vi "Save.vi"(0 "Digital in":refnum<vi>, 1 "new file path (Not A Path if cancelled) in":path, 2 "refnum in":refnum<file>, 5 "byte order (0:big-endian, network order)":T1(ring), 7 "Array":dbl[][](array[numeric]), 9 "Cluster":T2, 12 "Recording":bool, 13 "data":dbl[][](array[numeric]), 14 "Array 2":dbl[](array[numeric])) -> (4 "Byte Stream File out":refnum<file>, 6 "Save Path":path, 15 "new file path (Not A Path if cancelled)":path)   [LabVIEW 2018]
uses:
  <vilib>/Utility/file.llb/Write Delimited Spreadsheet (DBL).vi
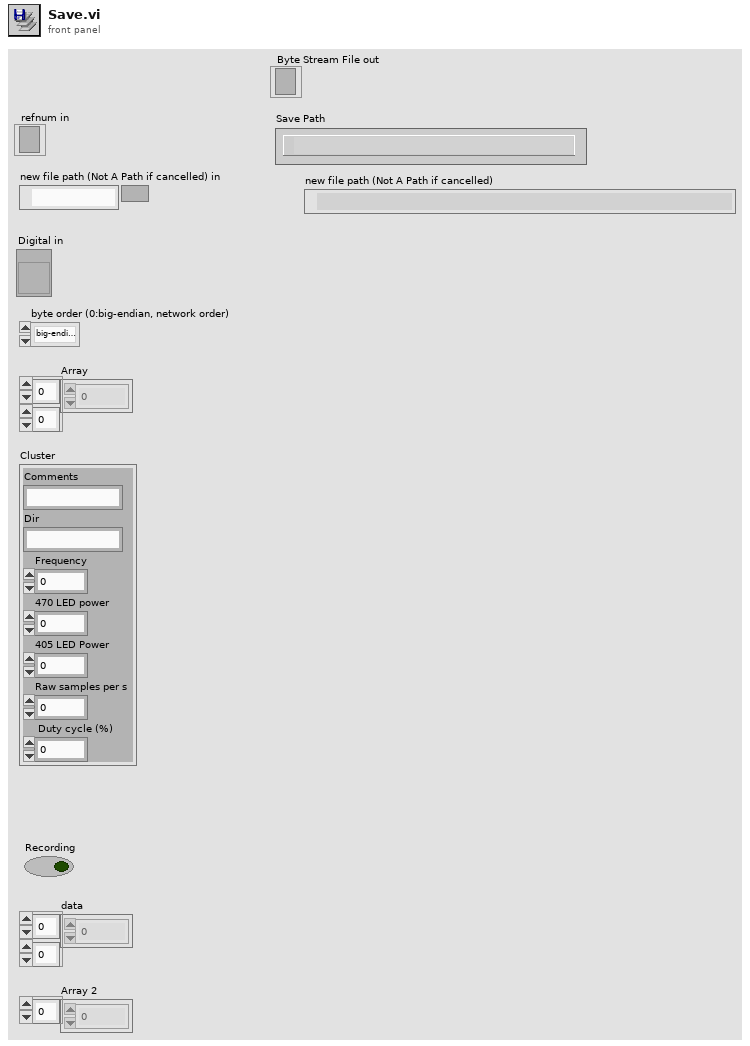
[diagram p1: front panel]
types:
  T1 = enum16{"big-endian, network order", "native, host order", "little-endian"}
  T2 = cluster{"Comments":string, "Dir":string, "Frequency":dbl, "470 LED power":dbl, "405 LED Power":dbl, "Raw samples per s":dbl, " Duty cycle (%)":dbl}
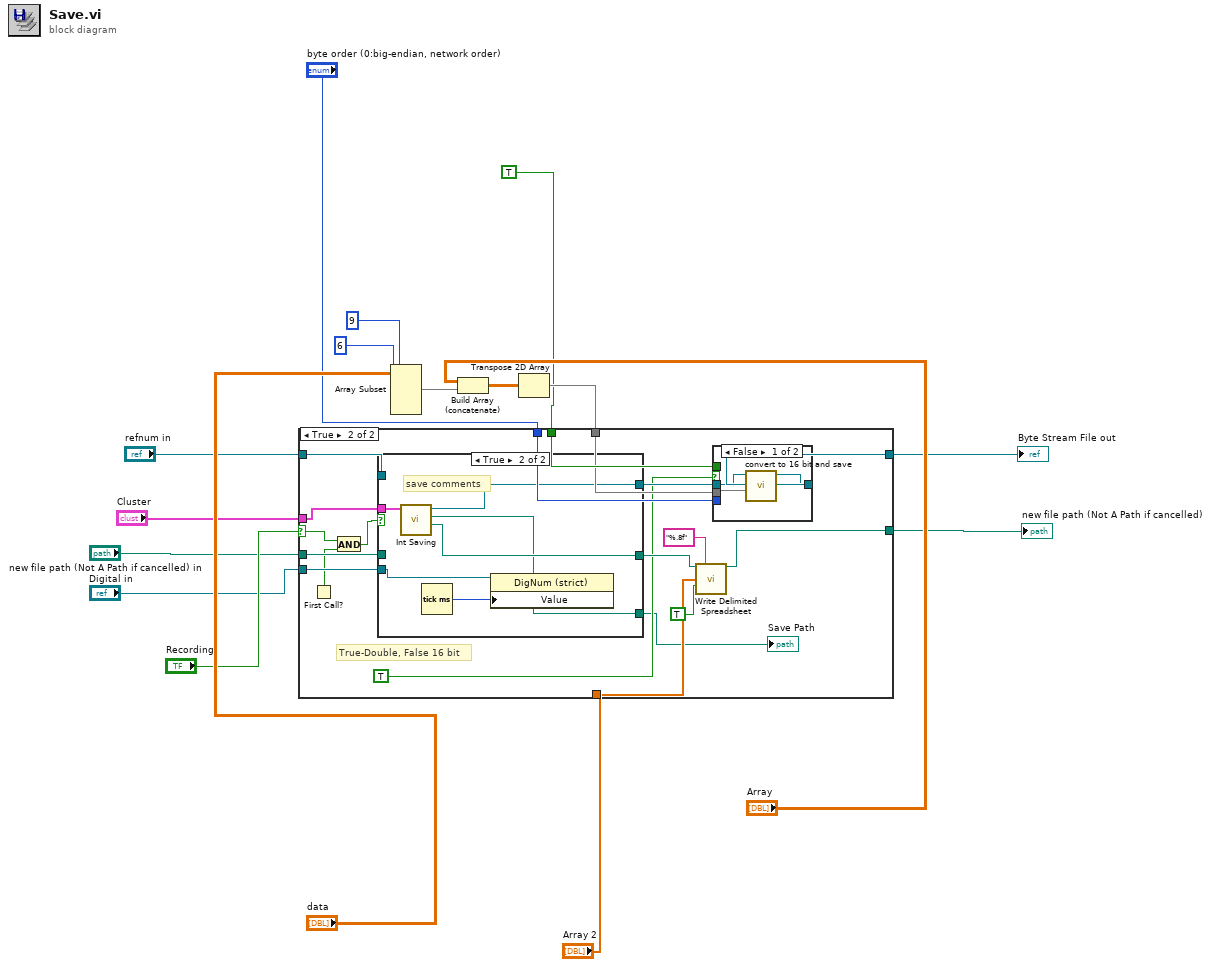
[diagram p0: block diagram]
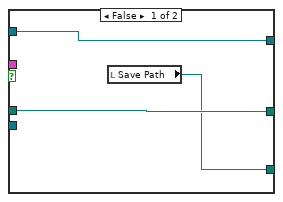
[diagram p3: hidden frame]
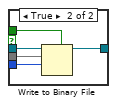
[diagram p4: hidden frame]
diagram:
  n1 = Array Subset(array="data", index (row)=9 ("disabled index (col)"), length (row)=6 ("length")) -> (w15:dbl[][])  [unwired: 2 in]
  n2 = Build Array (concatenate)("Array", w15) -> (w16:dbl[][])
  n3 = Transpose 2D Array(2D array=w16) -> (transposed array=w17:dbl[][])
  n4 = case shown="True" "Recording" {
    selector: "Recording" -> [_ w23]
    tunnel: "refnum in" -> [w19 w38]
    tunnel: [w19 w36] -> w5
    tunnel: TRUE -> [_ w35]
    tunnel: "byte order (0:big-endian, network order)" -> [_ w34]
    tunnel: "Array 2" -> [_ w31]
    tunnel: "Cluster" -> [_ w30]
    tunnel: [w18 w28] -> w1
    tunnel: "new file path (Not A Path if cancelled) in" -> [w18 w27]
    tunnel: w17 -> [_ w26]
    tunnel: "Digital in" -> [_ w24]
    frame False {
    }
    frame True {
      # "True-Double, False 16 bit"
      n5 = First Call?() -> (First Call?: T/F=w22:bool)
      n6 = And(x=w23, y=w22) -> (x .and. y?=w21:bool)
      n7 = case shown="True" w21 {
        tunnel: w38 -> [w41 _]
        tunnel: [w41 w47] -> w37
        tunnel: w30 -> [_ w46]
        tunnel: [w40 w45] -> w29
        tunnel: w27 -> [w40 _]
        tunnel: w24 -> [_ w43]
        tunnel: [w39 w42] -> w20
        frame False {
          n8 = local read "Save Path"() -> (w39:path)
        }
        frame True {
          # "save comments"
          n9 = call "Int Saving.vi"("Cluster"=w46) -> ("Data.txt"=w45:path, "created path"=w42:path, "Byte Stream File out"=w47:refnum<file>)  [unwired: 8 in]
          n10 = Tick Count (ms)() -> (millisecond timer value=w44:u32)
          n11 = property class="DigNum (strict)"(reference=w43, "Value"=w44) -> ()  [unwired: 1 in, 2 out]
        }
      }
      "Save Path" <- w20
      n12 = call-poly <vilib>:"Write Delimited Spreadsheet.vi"("file path (dialog if empty)"=w29, "format (%.3f)"="%.8f", "1D data"=w31, "append to file? (new file:F)"=TRUE) -> ("new file path (Not A Path if cancelled)"=w28:path)  [unwired: 10 in, 1 out]
      n13 = case shown="False" TRUE {
        tunnel: w37 -> [w49 w55]
        tunnel: [w48 w54] -> w36
        tunnel: w35 -> [_ w53]
        tunnel: w34 -> [_ w52]
        tunnel: w26 -> [w50 w51]
        frame False {
          n14 = call "convert to 16 bit and save.vi"("input array"=w50, "refnum in"=w49) -> ("refnum out"=w48:refnum<file>)  [unwired: 9 in]
        }
        frame True {
          n15 = Write to Binary File(file (use dialog)=w55, data=w51, 5:w53, 9:w52) -> (refnum out=w54:refnum<file>)  [unwired: 2 in, 2 out]
        }
      }
    }
  }
  "Byte Stream File out" <- w5
  "new file path (Not A Path if cancelled)" <- w1
